vi "Get Column Header Indexes.vi"(0 "Column Header Names":string[](array[string]), 11 "error in":errorcluster) -> (4 "Column Header Indices":i32[](array[numeric]), 6 "Column Header Exists?":bool[](array[boolean]), 15 "error out":errorcluster)   [LabVIEW 2023, in "RFCalAndFixtureCharact.Common.lvlib"]
uses:
  RFCalAndFixtureCharact.Common.lvlib
  Type Definitions/Dictionary Operation.ctl
  <vilib>/Utility/error.llb/Trim Whitespace One-Sided.vi
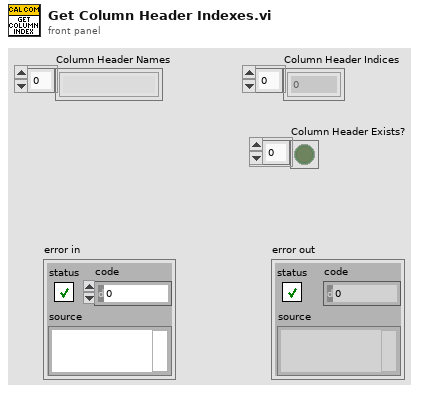
[diagram p1: front panel]
types:
  T1 = typedef "RFCalAndFixtureCharact.Common.lvlib/Dictionary Operation.ctl" = enum16{"Read", "Insert", "Remove", "Clear", "Get All", "Update"}
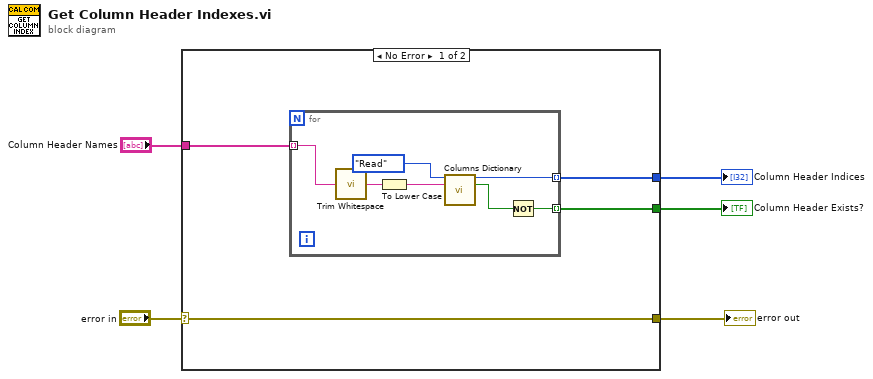
[diagram p0: block diagram]
diagram:
  n1 = case shown="No Error" "error in" {
    selector: "error in" -> [w9 w17]
    tunnel: [w9 w17] -> w4
    tunnel: "Column Header Names" -> [w8 _]
    tunnel: [w7 _] -> w2
    tunnel: [w6 _] -> w1
    frame No Error {
      n2 = for {
        tunnel: w8 -> [w14] mode=indexing
        tunnel: [w13] -> w7 mode=indexing
        tunnel: [w10] -> w6 mode=indexing
        n3 = call <vilib>:"Trim Whitespace.vi"("string"=w14) -> ("trimmed string"=w12:string)  [unwired: 1 in]
        n4 = To Lower Case(string=w12) -> (all lower case string=w15:string)
        n5 = call "Columns Dictionary.vi"("Action"=Dictionary_Operation."Read", "Column Header"=w15) -> ("Column Index"=w13:i32, "Column already included? / Column not found?"=w11:bool)  [unwired: 11 in, 1 out]
        n6 = Not(x=w11) -> (.not. x?=w10:bool)
      }
    }
    frame Error {
    }
  }
  "error out" <- w4
  "Column Header Indices" <- w2
  "Column Header Exists?" <- w1
